vi "GenerateHologram_josa.vi"(1 "Base":T1, 2 "Intensity Masking?":bool, 4 "Combined":T1) -> (0 "Array for SLM":u8[][](array[numeric]))   [LabVIEW 2015]
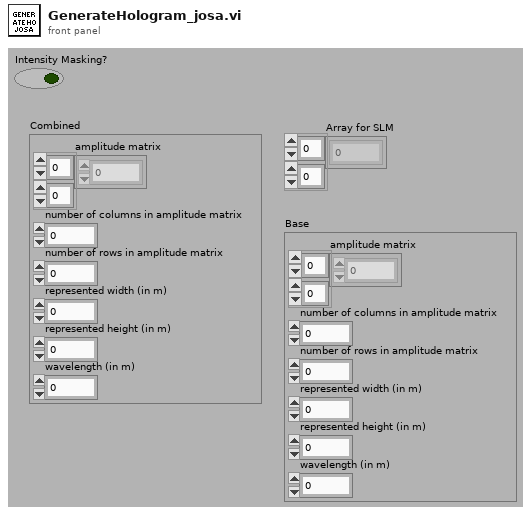
[diagram p1: front panel]
types:
  T1 = cluster{"amplitude matrix":cdb[][], "number of columns in amplitude matrix":i32, "number of rows in amplitude matrix":i32, "represented width (in m)":dbl, "represented height (in m)":dbl, "wavelength (in m)":dbl}
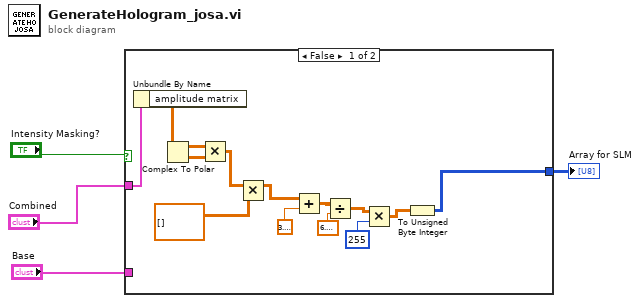
[diagram p0: block diagram]
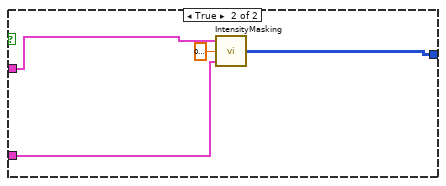
[diagram p2: hidden frame]
diagram:
  n1 = case shown="False" "Intensity Masking?" {
    tunnel: "Combined" -> [w9 w21]
    tunnel: [w11 w20] -> w2
    tunnel: "Base" -> [_ w19]
    frame False {
      n2 = Unbundle By Name(w9) -> ("amplitude matrix"=w8:cdb[][])
      n3 = Complex To Polar(r * e^(i*theta)=w8) -> (r=w7:dbl[][], theta=w6:dbl[][])
      n4 = Multiply(x=w7, y=w6) -> (x*y=w5:dbl[][])
      n5 = Multiply(x=w5, y=dbl[][] []) -> ()  [unwired: 1 out]
      n6 = Add(x=w5, y=3.141592653589793) -> (x+y=w14:dbl[][])
      n7 = Divide(x=w14, y=6.283185307179586) -> (x/y=w16:dbl[][])
      n8 = Multiply(x=w16, y=255) -> (x*y=w12:dbl[][])
      n9 = To Unsigned Byte Integer(number=w12) -> (unsigned 8bit integer=w11:u8[][])
    }
    frame True {
      n10 = call <userlib>:"IntensityMasking.vi"("Base"=w19, "Power in beam (1=max)"=0.9999999999999999, "Combined"=w21) -> ("Array"=w20:u8[][])
    }
  }
  "Array for SLM" <- w2
